vi "saveAsEvent.vi"(8 "error in (no error)":errorcluster, 11 "PixelflySettings in":refnum<class "PixelflySettings.lvclass">) -> (0 "error out":errorcluster, 3 "PixelflySettings out":refnum<class "PixelflySettings.lvclass">)   [LabVIEW 2009, in "Tools.lvlib" / "Settings.lvlib" / "PixelflySettings.lvclass"]
uses:
  PixelflySettings.lvclass
  PixelflySettings.lvclass/PixelflySettings.ctl
  SettingsViewer/settingsViewer.lvclass
  Filing.lvlib
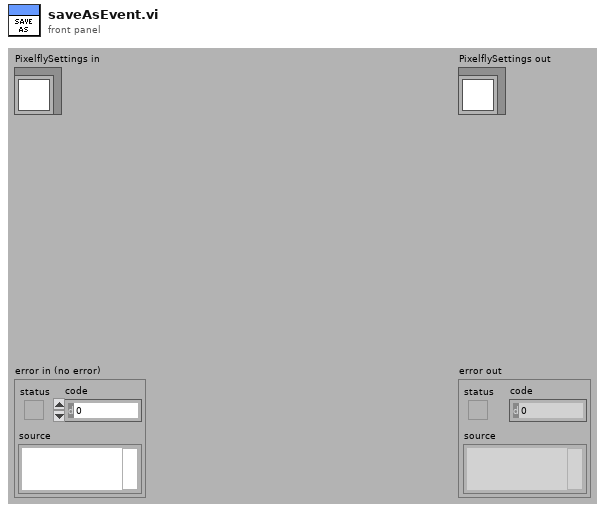
[diagram p1: front panel]
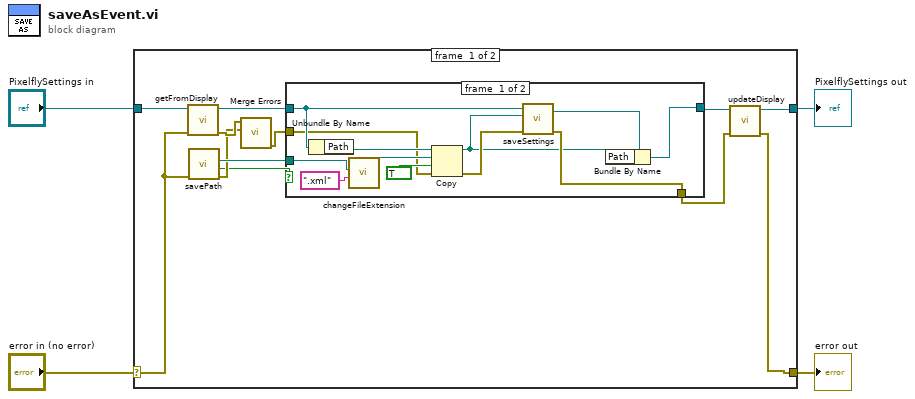
[diagram p0: block diagram]
diagram:
  n1 = case shown="No Error" "error in (no error)" {
    selector: "error in (no error)" -> [w13 w32]
    tunnel: [w5 w32] -> w3
    tunnel: [w7 w31] -> w1
    tunnel: "PixelflySettings in" -> [w16 w31]
    frame #0 {
      n2 = call "getFromDisplay.vi"("error in (no error)"=w13, "PixelflySettings in"=w16) -> ("error out"=w12:errorcluster, "PixelflySettings out"=w15:refnum<class "PixelflySettings.lvclass">)  [unwired: 8 in]
      n3 = call "savePath.vi"("error in (no error)"=w13) -> ("error out"=w11:errorcluster, "cancelled"=w10:bool, "Path out"=w14:path)  [unwired: 8 in]
      n4 = call <vilib>:"Merge Errors.vi"("error in 2 (no error)"=w11, "error in 1 (no error)"=w12) -> ("error out"=w9:errorcluster)  [unwired: 5 in]
      n5 = case shown="False" w10 {
        tunnel: [w21 w29] -> w6
        tunnel: w15 -> [w24 w30]
        tunnel: [w27 w30] -> w8
        tunnel: w14 -> [w25 _]
        tunnel: w9 -> [w19 w29]
        frame #0 {
          n6 = Unbundle By Name(w24) -> ("Path"=w23:path)
          n7 = call "changeFileExtension.vi"("extension"=".xml", "Path"=w25) -> ("Path out"=w22:path)  [unwired: 9 in]
          n8 = Copy(8:w19, 9:TRUE, 10:w22, 11:w23) -> (0:w18:errorcluster, 3:w17:path)  [unwired: 1 in, 1 out]
          n9 = call-dynamic "saveSettings.vi"("error in (no error)"=w18, "Path"=w17, "PixelflySettings in"=w24) -> ("error out"=w21:errorcluster, "PixelflySettings out"=w28:refnum<class "PixelflySettings.lvclass">)  [unwired: 7 in]
          n10 = Bundle By Name(cluster=w28, "Path"=w17) -> (w27:refnum<class "PixelflySettings.lvclass">)
        }
        frame #1 {
        }
      }
      n11 = call "updateDisplay.vi"("error in (no error)"=w6, "PixelflySettings in"=w8) -> ("error out"=w5:errorcluster, "PixelflySettings out"=w7:refnum<class "PixelflySettings.lvclass">)  [unwired: 8 in]
    }
    frame #1 {
    }
  }
  "error out" <- w3
  "PixelflySettings out" <- w1
